vi "Send Notification.vi"(8 "error in (no error)":errorcluster, 9 "Timeout":i32=-1, 10 "Notification":variant, 11 "RT FIFO I64 Notifier in":refnum<class "RT FIFO I64 Notifier.lvclass">) -> (0 "error out":errorcluster, 1 "Timeout?":bool, 3 "RT FIFO I64 Notifier out":refnum<class "RT FIFO I64 Notifier.lvclass">)   [LabVIEW 2022 SP3, in "RT FIFO I64 Notifier.lvclass"]
uses:
  RT FIFO I64 Notifier.lvclass
  RT FIFO I64 Notifier.lvclass/RT FIFO I64 Notifier.ctl
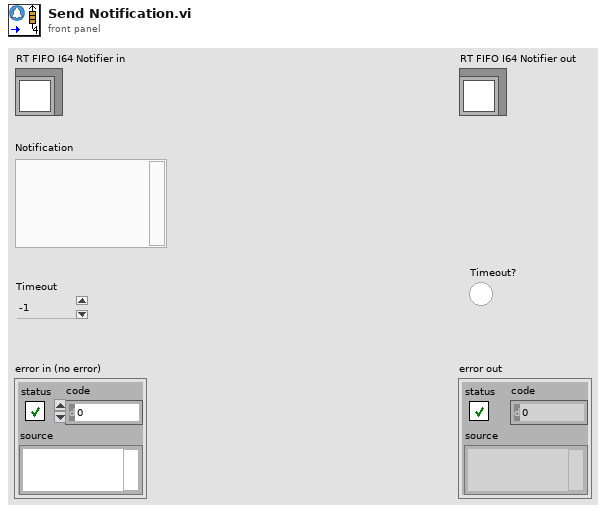
[diagram p1: front panel]
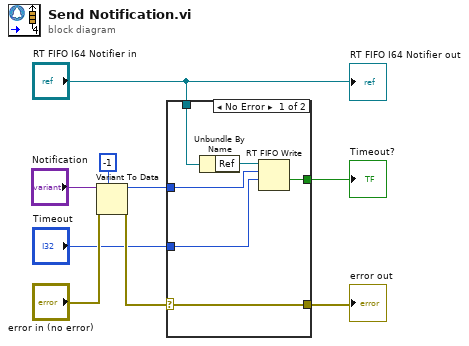
[diagram p0: block diagram]
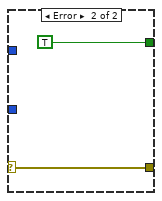
[diagram p2: hidden frame]
diagram:
  n1 = Variant To Data(error in="error in (no error)", type=i64 -1 ("Timeout"), Variant="Notification") -> (data=w4:i64, error out=w5:errorcluster)
  n2 = case shown="No Error" w5 {
    selector: w5 -> [w10 w17]
    tunnel: "RT FIFO I64 Notifier in" -> [w15 _]
    tunnel: w4 -> [w13 _]
    tunnel: "Timeout" -> [w12 _]
    tunnel: [w11 TRUE ("timed out?")] -> w2
    tunnel: [w10 w17] -> w1
    frame No Error {
      n3 = Unbundle By Name(w15) -> ("Ref"=w14:refnum<k33>)
      n4 = RT FIFO Write(0:w14, 1:w13, 2:w12) -> (10:w11:bool)  [unwired: 2 in, 3 out]
    }
    frame Error {
    }
  }
  "error out" <- w1
  "Timeout?" <- w2
  "RT FIFO I64 Notifier out" <- "RT FIFO I64 Notifier in"
